vi "Ramp.vi"(8 "error in (no error)":errorcluster, 10 "Max change (power / sec)":dbl, 11 "Joystick in":dbl) -> (0 "error out":errorcluster, 3 "Motor out":dbl)   [LabVIEW 2015]
doc: "Limits motor change to a certain change / time."
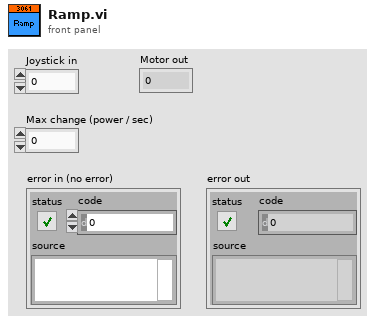
[diagram p1: front panel]
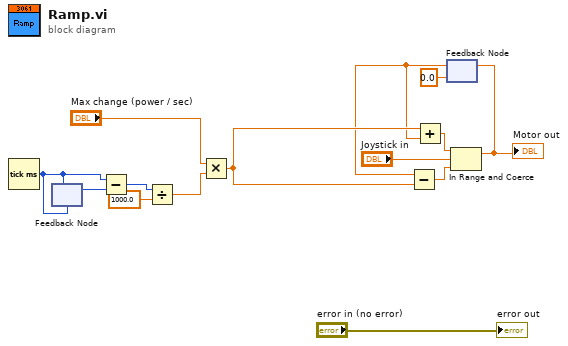
[diagram p0: block diagram]
diagram:
  n1 = Tick Count (ms)() -> (millisecond timer value=w14:u32)
  n2 = feedback-in #1(w14) -> ()
  n3 = feedback #1(w14) -> (w13:u32)
  n4 = Subtract(x=w14, y=w13) -> (x-y=w12:u32)
  n5 = Divide(x=w12, y=1000.0) -> (x/y=w10:dbl)
  n6 = Multiply(x="Max change (power / sec)", y=w10) -> (x*y=w8:dbl)
  n7 = feedback #2(0.0 ("Joystick in")) -> (w3:dbl)
  n8 = Subtract(x=w3, y=w8) -> (x-y=w6:dbl)
  n9 = Add(x=w8, y=w3) -> (x+y=w7:dbl)
  n10 = In Range and Coerce(upper limit=w7, x="Joystick in", lower limit=w6) -> (coerced(x)=w4:dbl)  [unwired: 1 out]
  "Motor out" <- w4
  n11 = feedback-in #2(w4) -> ()
  "error out" <- "error in (no error)"
